vi "CRYFlatten Post Processing.vi"(11 "Post-Processing":T1 {"user equation cluster"."Results axis" items=["x", "y", "z"]; "user equation cluster"."Input axis" items=["x", "y", "z"]; "user equation cluster"."Custom unit results array"."dB ref" format="%.2f"; "user equation cluster"."Custom unit input array"."dB ref" format="%.2f"; "Constant" format="%#.5p"; "Unary Operator" format="%10.0f"; "Custom unit info"."dB ref" format="%.2f"; "Sampling Rate" format="%#.2p"}) -> (3 "Post Processing flattened":string)   [LabVIEW 2013]
uses:
  Typedef Control/CRYPost Processing Cluster.ctl
  Typedef Control/CRYUser Equation Cluster.ctl
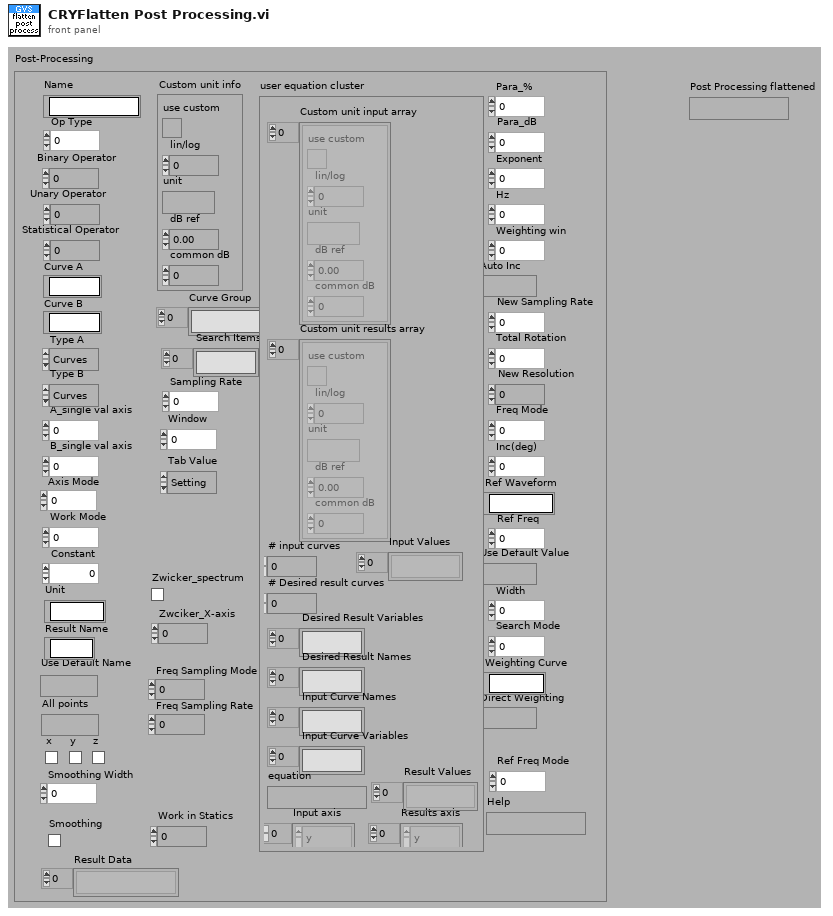
[diagram p1: front panel]
types:
  T1 = typedef "CRYPost Processing Cluster.ctl" = cluster{"Name":string, "Op Type":u16, "Curve A":string, "Curve B":string, "Axis Mode":u16, "Work Mode":u16, "Width":u16, "Weighting win":u16, "Search Mode":u16, "Freq Mode":u16, "New Sampling Rate":dbl, "Use Default Name":bool, "x":bool, "y":bool, "z":bool, "All points":bool, "A_single val axis":u16, "B_single val axis":u16, "Use Default Value":bool, "Result Name":string, "Smoothing Width":i32, "Window":u16, "Para_dB":sgl, "Para_%":sgl, "Exponent":sgl, "Hz":dbl, "Direct Weighting":bool, "Auto Inc":bool, "Inc(deg)":i32, "Total Rotation":i32, "Ref Freq Mode":u16, "Ref Waveform":string, "Sampling Rate":dbl, "Weighting Curve":string, "Ref Freq":dbl, "Curve Group":string[], "Search Items":string[], "Custom unit info":cluster{"use custom":bool, "lin/log":u16, "unit":string, "dB ref":dbl, "common dB":u16}, "Unit":string, "Type A":enum16{"Curves", "Values", "Results", "WFM"}, "Type B":enum16{"Curves", "Values", "Results", "WFM"}, "Unary Operator":u16, "Binary Operator":u16, "Statistical Operator":u16, "Constant ":dbl, "New Resolution":u16, "user equation cluster":T2, "Help":string, "Tab Value":enum32{"Setting", "Help"}, "Zwciker_X-axis":u16, "Zwicker_spectrum":bool, "Freq Sampling Mode":u16, "Freq Sampling Rate":dbl, "Smoothing":bool, "Work in Statics":u16, "Result Data":string[]}
  T2 = typedef "CRYUser Equation Cluster.ctl" = cluster{"Custom unit input array":cluster{"use custom":bool, "lin/log":u16, "unit":string, "dB ref":dbl, "common dB":u16}[], "Custom unit results array ":cluster{"use custom":bool, "lin/log":u16, "unit":string, "dB ref":dbl, "common dB":u16}[], "Desired Result Variables":string[], "Desired Result Names":string[], "Input Curve Names":string[], "Input Curve Variables":string[], "equation":string, "Input axis":u16[], "Results axis":u16[], "# input curves":i32, "# Desired result curves ":i32, "Input Values":string[], "Result Values":string[]}
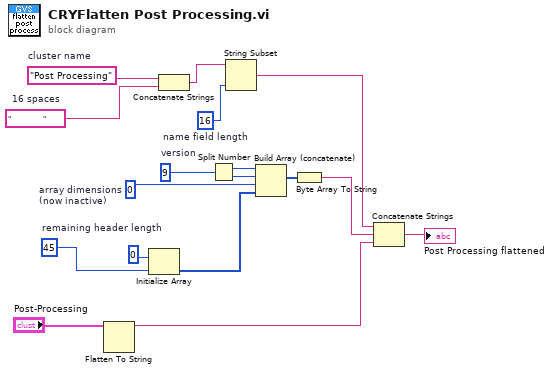
[diagram p0: block diagram]
diagram:
  w3 = u8 0  # array dimensions (now inactive)
  w6 = 16  # name field length
  w7 = "                "  # 16 spaces
  w8 = "Post Processing"  # cluster name
  w13 = 45  # remaining header length
  w17 = u16 9  # version
  n1 = Flatten To String(anything="Post-Processing") -> (data string=w2:string)  [unwired: 1 in, 4 out]
  n2 = Initialize Array(u8 0, w13) -> (w9:u8[])
  n3 = Concatenate Strings(w8, w7) -> (w5:string)
  n4 = Split Number(x=w17) -> (hi(x)=w16:u8, lo(x)=w15:u8)
  n5 = String Subset(string=w5, length (rest)=w6) -> (substring=w4:string)  [unwired: 1 out]
  n6 = Build Array (concatenate)(w16, w15, w3, w9) -> (w12:u8[])
  n7 = Byte Array To String(unsigned byte array=w12) -> (string=w10:string)
  n8 = Concatenate Strings(w4, w10, w2) -> (→"Post Processing flattened":string)
